vi "BYTE Size To WORD Size.vi"(1 "BYTE Size":u32) -> (0 "WORD Size":u32)   [LabVIEW 2010, in "KEYENCE LJ-X8000A.lvlib"]
uses:
  KEYENCE LJ-X8000A.lvlib
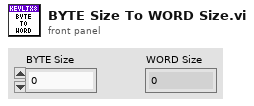
[diagram p1: front panel]
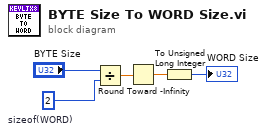
[diagram p0: block diagram]
diagram:
  w4 = u32 2  # sizeof(WORD)
  n1 = Divide(x="BYTE Size", y=w4) -> (x/y=w3:dbl)
  n2 = Round Toward -Infinity(1:w3) -> (0:w2:dbl)
  n3 = To Unsigned Long Integer(number=w2) -> (unsigned 32bit integer=→"WORD Size":u32)
